vi "Digital Pin State to String.vi"(7 "Pin State":T1 items=["0"=0, "1"=1, "L"=3, "H"=4, "X"=5, "M"=6, "V"=7, "D"=8, "E"=9, "Not A Pin State"=254, "Pin State Not Acquired"=255]) -> (8 "String":string)   [LabVIEW 2019]
uses:
  <instrlib>/niDigital/niDigital.llb/niDigital Pin State.ctl
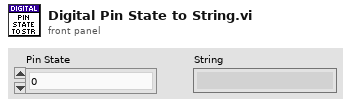
[diagram p1: front panel]
types:
  T1 = typedef "niDigital Pin State.ctl" = u8
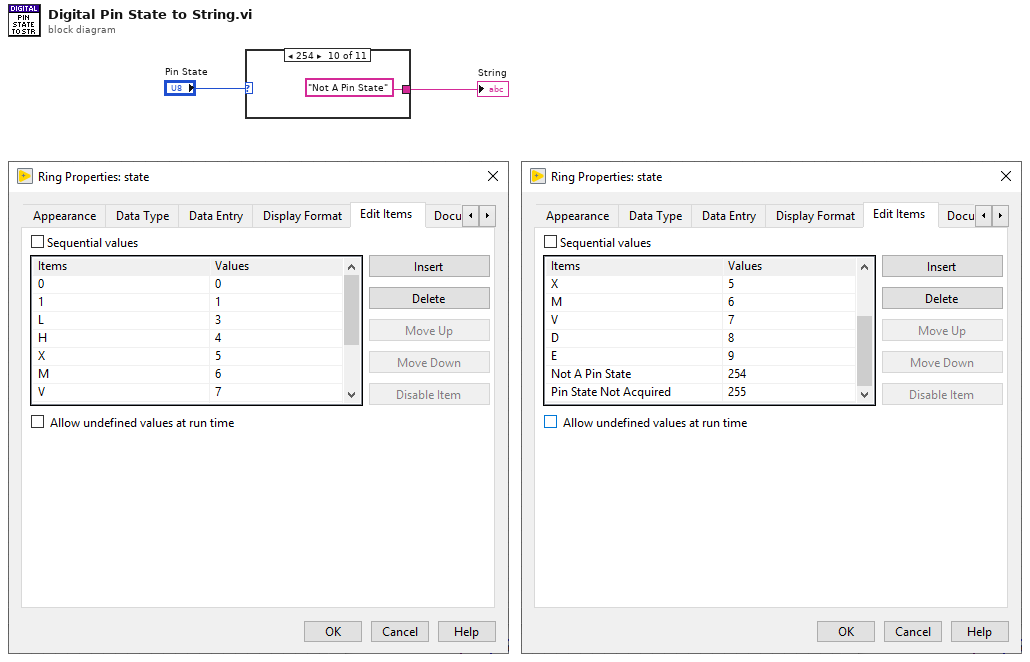
[diagram p0: block diagram]
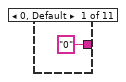
[diagram p2: hidden frame]
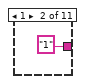
[diagram p3: hidden frame]
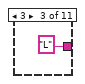
[diagram p4: hidden frame]
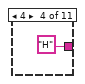
[diagram p5: hidden frame]
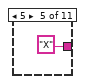
[diagram p6: hidden frame]
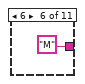
[diagram p7: hidden frame]
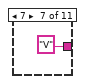
[diagram p8: hidden frame]
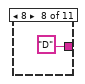
[diagram p9: hidden frame]
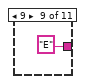
[diagram p10: hidden frame]
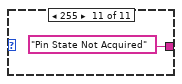
[diagram p11: hidden frame]
diagram:
  n1 = case shown="254" "Pin State" {
    tunnel: ["0" "1" "L" "H" "X" "M" "V" "D" "E" "Not A Pin State" "Pin State Not Acquired"] -> w2
    frame 0, Default {
    }
    frame 1 {
    }
    frame 3 {
    }
    frame 4 {
    }
    frame 5 {
    }
    frame 6 {
    }
    frame 7 {
    }
    frame 8 {
    }
    frame 9 {
    }
    frame 254 {
    }
    frame 255 {
    }
  }
  "String" <- w2
